vi "13 Case Structures.vi"() -> ()   [LabVIEW 2019]
uses:
  _Subs/OpenDiagram/OpenDiag.xctl
panel:
  in  "OpenDiag":refnum<vi>(xcontrol)
  out "Status":string
  in  "Boolean":bool
  in  "Enum":enum16{"Foot", "Bike", "Car", "Plane"}(ring)=enum."Plane"
  out "Speed 2":string
  out "Speed":string
  out "info":string
  in  "Ring":u16(ring)=3 items=["Foot", "Bike", "Car", "Plane"]
  in  "Numeric":i32=5
  # "13 Case Structures\nThis code demonstrates different ways of using the case statement\n\nInstructions:\n1. Hit the Run arrow and see the code execute"
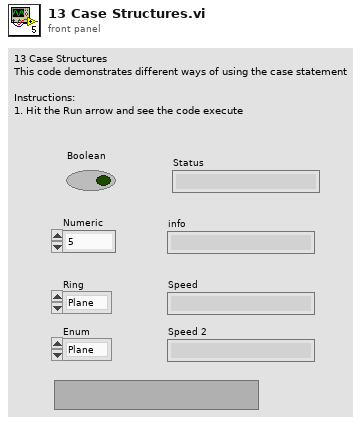
[diagram p1: front panel]
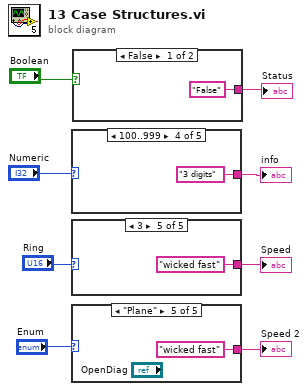
[diagram p0: block diagram]
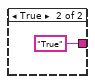
[diagram p2: hidden frame]
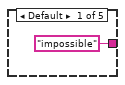
[diagram p3: hidden frame]
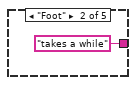
[diagram p4: hidden frame]
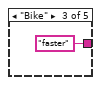
[diagram p5: hidden frame]
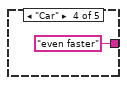
[diagram p6: hidden frame]
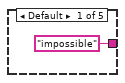
[diagram p7: hidden frame]
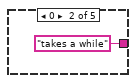
[diagram p8: hidden frame]
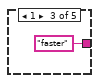
[diagram p9: hidden frame]
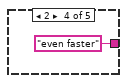
[diagram p10: hidden frame]
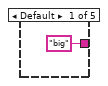
[diagram p11: hidden frame]
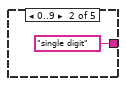
[diagram p12: hidden frame]
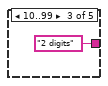
[diagram p13: hidden frame]
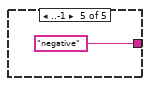
[diagram p14: hidden frame]
diagram:
  n1 = case shown="100..999" "Numeric" {
    tunnel: ["big" "single digit" "2 digits" "3 digits" "negative"] -> w7
    frame Default {
    }
    frame 0..9 {
    }
    frame 10..99 {
    }
    frame 100..999 {
    }
    frame ..-1 {
    }
  }
  "info" <- w7
  n2 = case shown="3" "Ring" {
    tunnel: ["impossible" "takes a while" "faster" "even faster" "wicked fast"] -> w5
    frame Default {
    }
    frame 0 {
    }
    frame 1 {
    }
    frame 2 {
    }
    frame 3 {
    }
  }
  "Speed" <- w5
  n3 = case shown="\"Plane\"" "Enum" {
    tunnel: ["impossible" "takes a while" "faster" "even faster" "wicked fast"] -> w4
    frame Default {
    }
    frame "Foot" {
    }
    frame "Bike" {
    }
    frame "Car" {
    }
    frame "Plane" {
    }
  }
  "Speed 2" <- w4
  n4 = case shown="False" "Boolean" {
    tunnel: ["False" "True"] -> w1
    frame False {
    }
    frame True {
    }
  }
  "Status" <- w1
